vi "Calculate Osculating Terms.vi"(7 "tau":dbl, 11 "ABC Coefficient Array":dbl[][](array[numeric])) -> (2 "Series Sum":dbl=114172100469.83818, 3 "Series Terms":dbl[](array[numeric])=[-0.6536436208636119, -1.9799849932008908, -0.4161468365471424] format="%#_12f")   [LabVIEW 2015]
panel:
  # "From Meeus page 218, (just below equation 32.1\n\nSeries Terms = A cos (B + Ct)\n\nB and C expressed in Radians\nA coefficients are in units of 10^-8 radians in the case of longitude\nand 10^-8 AU for the radius vector"
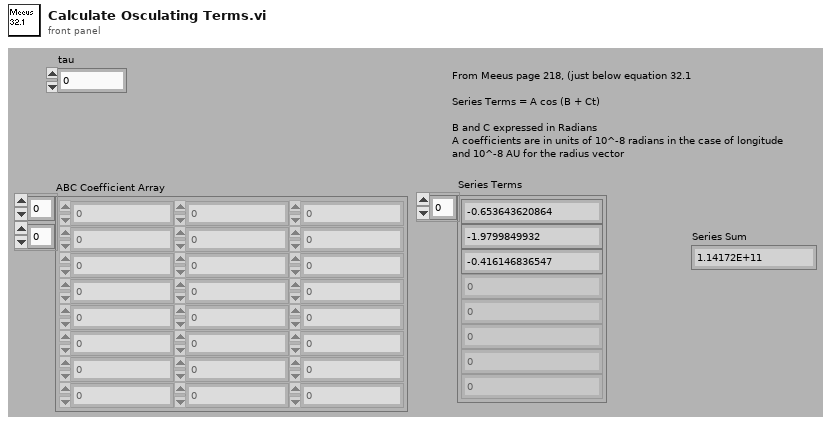
[diagram p1: front panel]
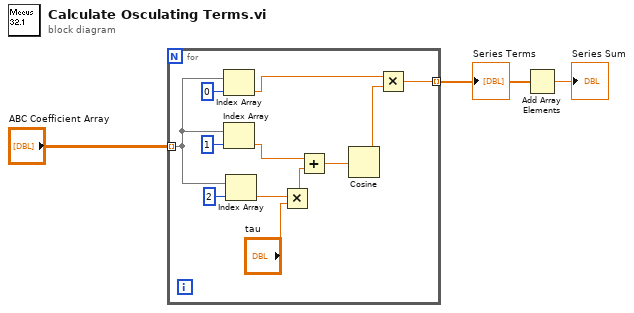
[diagram p0: block diagram]
diagram:
  n1 = for {
    tunnel: "ABC Coefficient Array" -> [w12] mode=indexing
    tunnel: [w4] -> w3 mode=indexing
    n2 = Index Array(array=w12, index=0) -> (element=w5:dbl)
    n3 = Index Array(array=w12, index=1) -> (element=w8:dbl)
    n4 = Index Array(array=w12, index=2) -> (element=w11:dbl)
    n5 = Multiply(x=w11, y="tau") -> (x*y=w9:dbl)
    n6 = Add(x=w8, y=w9) -> (x+y=w7:dbl)
    n7 = Cosine(x=w7) -> (cos(x)=w6:dbl)
    n8 = Multiply(x=w5, y=w6) -> (x*y=w4:dbl)
  }
  "Series Terms" <- w3
  n9 = Add Array Elements(numeric array=w3) -> (sum=→"Series Sum":dbl)
